vi "StartHeading.vi"(9 "Block Array":dbl[][](array[numeric])=[[3.0, 13.0, 345.0, 1495.0, 0.0, 0.0, 0.66125, 1.495, 1.5707963267948966, 100.0], [18.0, 8.0, 2070.0, 920.0, 0.0, 0.0, 1.75375, 0.92, -1.5707963267948966, 100.0], [13.0, 4.0, 1495.0, 460.0, 0.0, 0.0, 1.495, 0.77625, 3.141592653589793, 100.0]], 11 "Start POS":dbl[](array[numeric])=[1.385901420724191, 1.2768028414483816, -2.819842099193151]) -> (1 "Heading rad back":dbl, 2 "block array out":dbl[][](array[numeric]))   [LabVIEW 2018]
uses:
  cebfb251-3405-4e07-ab95-7f58c85577fe.vi
  <vilib>/Array/Sort 2D Array - Pop Stack.vi
  <vilib>/Array/Sort 2D Array - Push Stack.vi
  cebfb251-3405-4e07-ab95-7f58c85577fe.vi/ae38da9d-179d-4755-a5db-9122b6f68427.vi
  cebfb251-3405-4e07-ab95-7f58c85577fe.vi/bbdec304-1773-4e0c-8f0f-3f3b91127dab.vi
panel:
  out "haha":dbl[][](array[numeric])
  out "FIX ARRAY":dbl[][](array[numeric])
  out "Target theta":dbl
  out "included deg":dbl
  out "InRange":bool
  out "In deg":dbl
  out "Out deg":dbl
  out "Target deg":dbl
  out "Heading rad":dbl
  out "start":dbl
  out "Target d":dbl[](array[numeric])
  out "Array":dbl[](array[numeric])
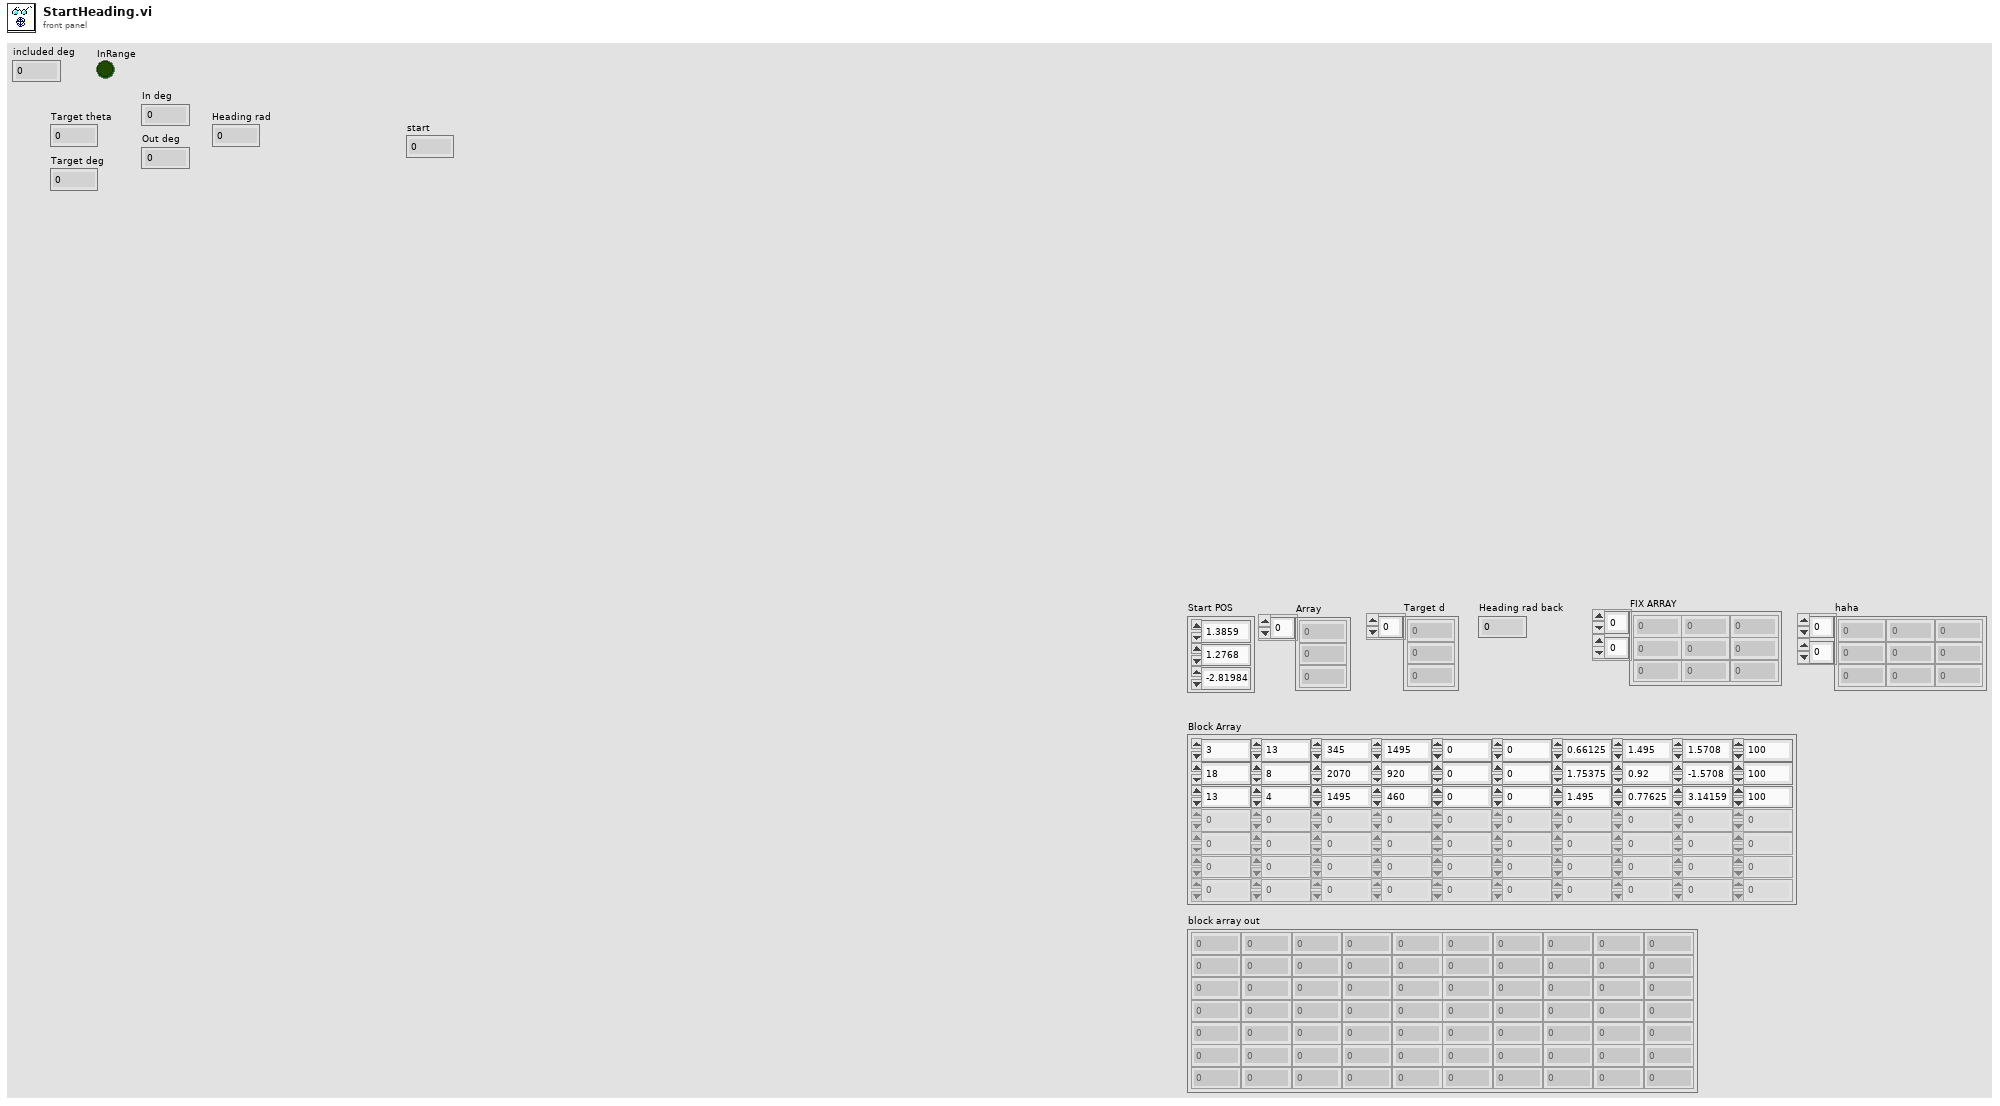
[diagram p1: front panel]
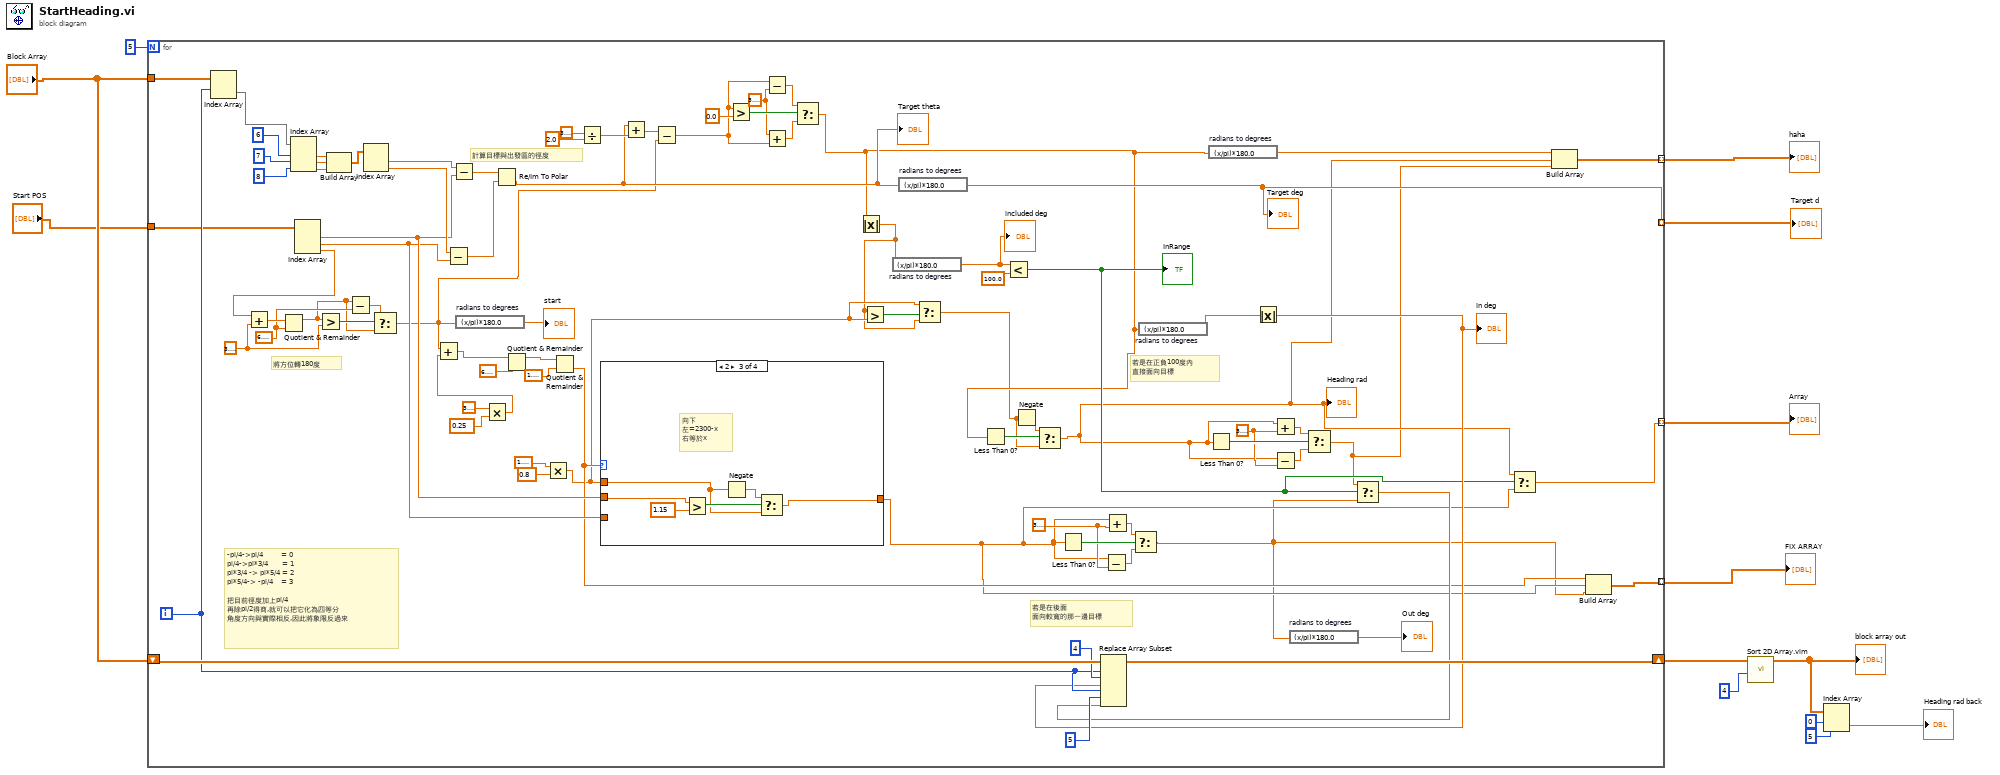
[diagram p0: block diagram]
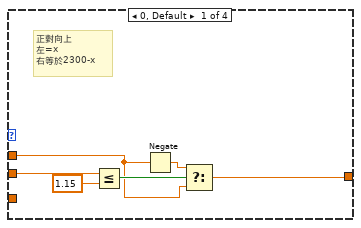
[diagram p2: hidden frame]
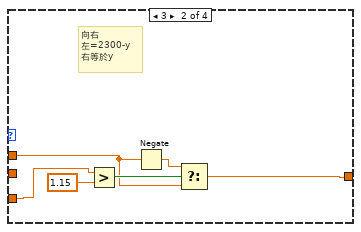
[diagram p3: hidden frame]
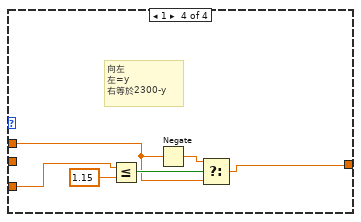
[diagram p4: hidden frame]
diagram:
  n1 = for {
    N: 5 -> [_]
    tunnel: "Block Array" -> [w63]
    shift-right: [w58] -> w7
    shift-left: "Block Array" -> [w62]
    tunnel: [w34] -> w6 mode=indexing
    tunnel: [w50] -> w4 mode=indexing
    tunnel: "Start POS" -> [w32]
    tunnel: [w29] -> w5 mode=indexing
    tunnel: [w15] -> w3 mode=indexing
    i -> [w60]
    w35 = 3.141592653589793
    w41 = 3.141592653589793
    w75 = 6.283185307179586
    w78 = 3.141592653589793
    w26 = 3.141592653589793
    # "將方位轉180度"
    # "若是在後面\n面向較寬的那一邊目標"
    # "若是在正負100度內\n直接面向目標"
    # "-pi/4->pi/4         = 0\npi/4->pi*3/4       = 1\npi*3/4 -> pi*5/4 = 2\npi*5/4-> -pi/4    = 3\n\n把目前徑度加上pi/4\n再除pi/2得商,就可以把它化為四等分\n角度方向與實際相反,因此將象限反過來"
    # "計算目標與出發區的徑度"
    n2 = Index Array(array=w63, index (row)=w60) -> (element=w68:dbl[])  [unwired: 1 in]
    n3 = Index Array(array=w68, index #1=6 ("index"), index #2=7 ("index"), index #3=8 ("index")) -> (element #1=w67:dbl, element #2=w66:dbl, element #3=w65:dbl)
    n4 = Index Array(array=w32) -> (element #1=w86:dbl, element #2=w85:dbl, element #3=w28:dbl)  [unwired: 3 in]
    n5 = Add(x=w28, y=w78) -> (x+y=w79:dbl)
    n6 = Quotient & Remainder(x=w79, y=w75) -> (x-y*floor(x/y)=w74:dbl)  [unwired: 1 out]
    n7 = Greater?(x=w74, y=w78) -> (0:w77:bool)
    n8 = Build Array(w67, w66, w65) -> (w64:dbl[])
    n9 = Subtract(x=w74, y=w75) -> (x-y=w76:dbl)
    n10 = Index Array(array=w64) -> (element #1=w95:dbl, element #2=w94:dbl)  [unwired: 2 in]
    n11 = Select(t=w76, s=w77, f=w74) -> (s? t:f=w46:dbl)
    n12 = Subtract(x=w94, y=w85) -> (x-y=w57:dbl)
    n13 = Subtract(x=w95, y=w86) -> (x-y=w56:dbl)
    n14 = expression code="(x/pi)*180.0" "radians to degrees"(w46) -> (→"start":dbl)
    n15 = Multiply(x=3.141592653589793, y=0.25) -> (x*y=w88:dbl)
    n16 = Add(x=w46, y=w88) -> (x+y=w27:dbl)
    n17 = Re/Im To Polar(2:w57, 3:w56) -> (0:w49:dbl)  [unwired: 1 out]
    "Target theta" <- w49
    n18 = Quotient & Remainder(x=w27, y=6.283185307179586) -> (x-y*floor(x/y)=w91:dbl)  [unwired: 1 out]
    n19 = Multiply(x=1.5707963267948966, y=0.8) -> (x*y=w23:dbl)
    n20 = Quotient & Remainder(x=w91, y=1.5707963267948966) -> (floor(x/y)=w31:dbl)  [unwired: 1 out]
    n21 = Divide(x=3.141592653589793, y=2.0) -> (x/y=w53:dbl)
    n22 = case shown="2" w31 {
      tunnel: w86 -> [w101 _ w111 _]
      tunnel: w85 -> [_ w105 _ w117]
      tunnel: [w98 w104 w110 w116] -> w30
      tunnel: w23 -> [w96 w102 w108 w114]
      frame 0, Default {
        # "正對向上\n左=x\n右等於2300-x"
        n23 = Less Or Equal?(x=w101, y=1.15) -> (x <= y?=w99:bool)
        n24 = Negate(x=w96) -> (-x=w97:dbl)
        n25 = Select(t=w97, s=w99, f=w96) -> (s? t:f=w98:dbl)
      }
      frame 3 {
        # "向右\n左=2300-y\n右等於y"
        n26 = Greater?(x=w105, y=1.15) -> (0:w106:bool)
        n27 = Negate(x=w102) -> (-x=w103:dbl)
        n28 = Select(t=w103, s=w106, f=w102) -> (s? t:f=w104:dbl)
      }
      frame 2 {
        # "向下\n左=2300-x\n右等於x"
        n29 = Greater?(x=w111, y=1.15) -> (0:w112:bool)
        n30 = Negate(x=w108) -> (-x=w109:dbl)
        n31 = Select(t=w109, s=w112, f=w108) -> (s? t:f=w110:dbl)
      }
      frame 1 {
        # "向左\n左=y\n右等於2300-y"
        n32 = Less Or Equal?(x=w117, y=1.15) -> (x <= y?=w118:bool)
        n33 = Negate(x=w114) -> (-x=w115:dbl)
        n34 = Select(t=w115, s=w118, f=w114) -> (s? t:f=w116:dbl)
      }
    }
    n35 = Add(x=w49, y=w53) -> (x+y=w48:dbl)
    n36 = Subtract(x=w48, y=w46) -> (x-y=w40:dbl)
    n37 = Greater?(x=w40, y=0.0) -> (0:w44:bool)
    n38 = Subtract(x=w40, y=w41) -> (x-y=w43:dbl)
    n39 = Add(x=w41, y=w40) -> (x+y=w42:dbl)
    n40 = Select(t=w43, s=w44, f=w42) -> (s? t:f=w21:dbl)
    n41 = Absolute Value(x=w21) -> (abs(x)=w14:dbl)
    n42 = Greater?(x=w14, y=w23) -> (0:w24:bool)
    n43 = expression code="(x/pi)*180.0" "radians to degrees"(w14) -> (w84:dbl)
    "included deg" <- w84
    n44 = expression code="(x/pi)*180.0" "radians to degrees"(w49) -> (w50:dbl)
    "Target deg" <- w50
    n45 = Select(t=w23, s=w24, f=w14) -> (s? t:f=w19:dbl)
    n46 = Less Than 0?(x=w21) -> (x < 0?=w20:bool)
    n47 = Less?(x=w84, y=100.0) -> (x < y?=w33:bool)
    "InRange" <- w33
    n48 = Negate(x=w19) -> (-x=w22:dbl)
    n49 = Select(t=w22, s=w20, f=w19) -> (s? t:f=w17:dbl)
    "Heading rad" <- w17
    n50 = Less Than 0?(x=w30) -> (x < 0?=w38:bool)
    n51 = Subtract(x=w30, y=w35) -> (x-y=w37:dbl)
    n52 = Add(x=w30, y=w35) -> (x+y=w36:dbl)
    n53 = Select(t=w36, s=w38, f=w37) -> (s? t:f=w25:dbl)
    n54 = expression code="(x/pi)*180.0" "radians to degrees"(w21) -> (w52:dbl)
    n55 = expression code="(x/pi)*180.0" "radians to degrees"(w21) -> (w18:dbl)
    n56 = Less Than 0?(x=w17) -> (x < 0?=w82:bool)
    n57 = Absolute Value(x=w52) -> (abs(x)=w51:dbl)
    "In deg" <- w51
    n58 = Add(x=w17, y=w26) -> (x+y=w81:dbl)
    n59 = Subtract(x=w17, y=w26) -> (x-y=w80:dbl)
    n60 = expression code="(x/pi)*180.0" "radians to degrees"(w25) -> (→"Out deg":dbl)
    n61 = Select(t=w81, s=w82, f=w80) -> (s? t:f=w16:dbl)
    n62 = Select(t=w16, s=w33, f=w25) -> (s? t:f=w39:dbl)
    n63 = Replace Array Subset(array=w62, new element #1=w51, index (row) #1=w60, index (col) #1=4 ("disabled index (col)"), new element #2=w39, index (row) #2=w60, index (col) #2=5 ("disabled index (col)")) -> (w58:dbl[][])
    n64 = Select(t=w17, s=w33, f=w30) -> (s? t:f=w34:dbl)
    n65 = Build Array(w18, w17, w16) -> (w15:dbl[])
    n66 = Build Array(w31, w30, w25) -> (w29:dbl[])
  }
  "Array" <- w6
  "Target d" <- w4
  "FIX ARRAY" <- w5
  "haha" <- w3
  n67 = call "Sort 2D Array.vim"("index"=4, "2D array"=w7) -> ("sorted 2D array"=w12:dbl[][])  [unwired: 8 in, 1 out]
  "block array out" <- w12
  n68 = Index Array(array=w12, index (row)=0, index (col)=5 ("disabled index (col)")) -> (element=→"Heading rad back":dbl)
